vi "MFR Flow to SP.vi"(10 "MFC SPs":dbl[](array[numeric])) -> (2 "MFC array":dbl[](array[numeric]))   [LabVIEW 2014]
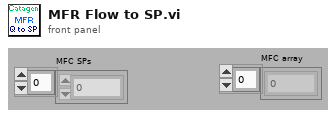
[diagram p1: front panel]
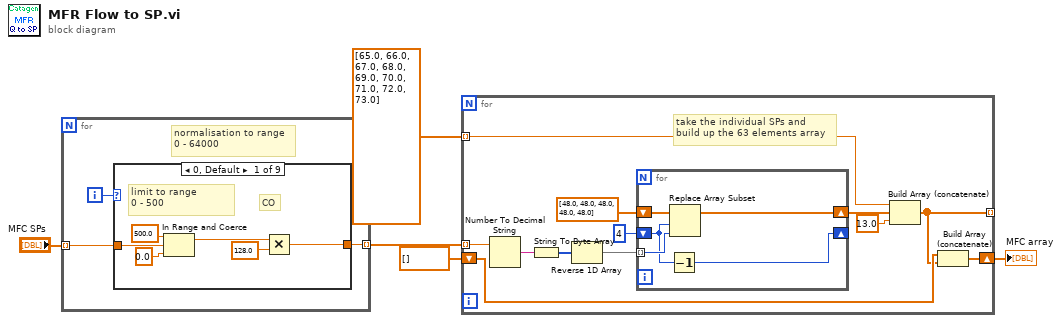
[diagram p0: block diagram]
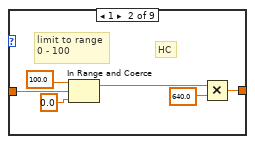
[diagram p2: hidden frame]
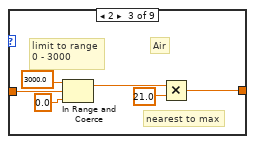
[diagram p3: hidden frame]
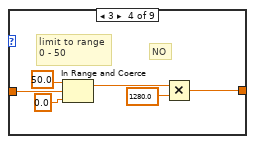
[diagram p4: hidden frame]
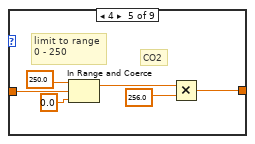
[diagram p5: hidden frame]
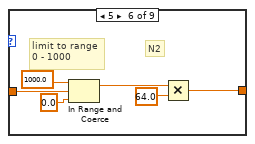
[diagram p6: hidden frame]
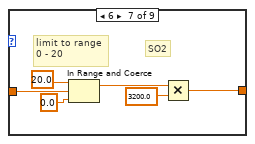
[diagram p7: hidden frame]
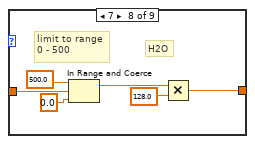
[diagram p8: hidden frame]
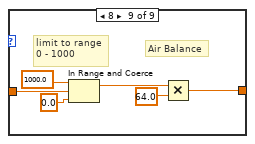
[diagram p9: hidden frame]
diagram:
  n1 = for {
    tunnel: "MFC SPs" -> [w7] mode=indexing
    tunnel: [w6] -> w1 mode=indexing
    i -> [w8]
    # "normalisation to range\n0 - 64000"
    n2 = case shown="0, Default" w8 {
      tunnel: w7 -> [w10 w17 w22 w28 w34 w40 w46 w52 w58]
      tunnel: [w13 w19 w25 w31 w37 w43 w49 w55 w61] -> w6
      frame 0, Default {
        # "CO"
        # "limit to range\n0 - 500"
        n3 = In Range and Coerce(upper limit=500.0, x=w10, lower limit=0.0) -> (coerced(x)=w9:dbl)  [unwired: 1 out]
        n4 = Multiply(x=w9, y=128.0) -> (x*y=w13:dbl)
      }
      frame 1 {
        # "HC"
        # "limit to range\n0 - 100"
        n5 = In Range and Coerce(upper limit=100.0, x=w17, lower limit=0.0) -> (coerced(x)=w15:dbl)  [unwired: 1 out]
        n6 = Multiply(x=w15, y=640.0) -> (x*y=w19:dbl)
      }
      frame 2 {
        # "nearest to max"
        # "Air"
        # "limit to range\n0 - 3000"
        n7 = In Range and Coerce(upper limit=3000.0, x=w22, lower limit=0.0) -> (coerced(x)=w21:dbl)  [unwired: 1 out]
        n8 = Multiply(x=w21, y=21.0) -> (x*y=w25:dbl)
      }
      frame 3 {
        # "NO"
        # "limit to range\n0 - 50"
        n9 = In Range and Coerce(upper limit=50.0, x=w28, lower limit=0.0) -> (coerced(x)=w27:dbl)  [unwired: 1 out]
        n10 = Multiply(x=w27, y=1280.0) -> (x*y=w31:dbl)
      }
      frame 4 {
        # "CO2"
        # "limit to range\n0 - 250"
        n11 = In Range and Coerce(upper limit=250.0, x=w34, lower limit=0.0) -> (coerced(x)=w33:dbl)  [unwired: 1 out]
        n12 = Multiply(x=w33, y=256.0) -> (x*y=w37:dbl)
      }
      frame 5 {
        # "N2"
        # "limit to range\n0 - 1000"
        n13 = In Range and Coerce(upper limit=1000.0, x=w40, lower limit=0.0) -> (coerced(x)=w39:dbl)  [unwired: 1 out]
        n14 = Multiply(x=w39, y=64.0) -> (x*y=w43:dbl)
      }
      frame 6 {
        # "SO2"
        # "limit to range\n0 - 20"
        n15 = In Range and Coerce(upper limit=20.0, x=w46, lower limit=0.0) -> (coerced(x)=w45:dbl)  [unwired: 1 out]
        n16 = Multiply(x=w45, y=3200.0) -> (x*y=w49:dbl)
      }
      frame 7 {
        # "H2O"
        # "limit to range\n0 - 500"
        n17 = In Range and Coerce(upper limit=500.0, x=w52, lower limit=0.0) -> (coerced(x)=w51:dbl)  [unwired: 1 out]
        n18 = Multiply(x=w51, y=128.0) -> (x*y=w55:dbl)
      }
      frame 8 {
        # "Air Balance"
        # "limit to range\n0 - 1000"
        n19 = In Range and Coerce(upper limit=1000.0, x=w58, lower limit=0.0) -> (coerced(x)=w57:dbl)  [unwired: 1 out]
        n20 = Multiply(x=w57, y=64.0) -> (x*y=w61:dbl)
      }
    }
  }
  n21 = for {
    tunnel: dbl[] [65.0, 66.0, 67.0, 68.0, 69.0, 70.0, 71.0, 72.0, 73.0] -> [w69] mode=indexing
    tunnel: [w65] -> _ mode=indexing
    shift-right: [w64] -> w3
    shift-left: dbl[] [] -> [w66]
    tunnel: w1 -> [w63] mode=indexing
    # "take the individual SPs and \nbuild up the 63 elements array"
    n22 = Number To Decimal String(number=w63) -> (decimal integer string=w70:string)  [unwired: 1 in]
    n23 = String To Byte Array(string=w70) -> (unsigned byte array=w73:u8[])
    n24 = Reverse 1D Array(array=w73) -> (reversed array=w74:u8[])
    n25 = for {
      tunnel: w74 -> [w77] mode=indexing
      shift-right: [w76] -> _
      shift-left: u8 4 -> [w75]
      shift-right: [w78] -> w67
      shift-left: dbl[] [48.0, 48.0, 48.0, 48.0, 48.0] -> [w79]
      n26 = Decrement(x=w75) -> (x-1=w76:u8)
      n27 = Replace Array Subset(array=w79, new element=w77, index=w75) -> (w78:dbl[])
    }
    n28 = Build Array (concatenate)(w69, w67, 13.0) -> (w65:dbl[])
    n29 = Build Array (concatenate)(w66, w65) -> (w64:dbl[])
  }
  "MFC array" <- w3
